vi "GUNSC_LibGetMaxAmps.vi"(8 "error in (no error)":errorcluster) -> (0 "error out":errorcluster, 2 "max amps":i32)   [LabVIEW 2014]
uses:
  public/c/lib/libunsc.so
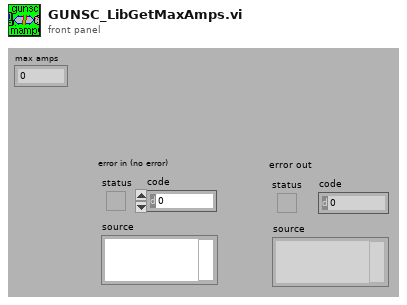
[diagram p1: front panel]
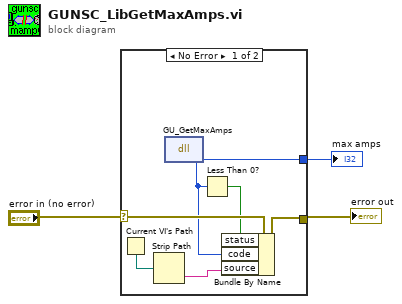
[diagram p0: block diagram]
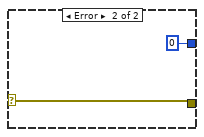
[diagram p2: hidden frame]
diagram:
  n1 = case shown="No Error" "error in (no error)" {
    selector: "error in (no error)" -> [w9 w11]
    tunnel: [w7 0] -> w3
    tunnel: [w4 w11] -> w1
    frame No Error {
      n2 = Current VI's Path() -> (path=w6:path)
      n3 = Strip Path(path=w6) -> (name=w5:string)  [unwired: 1 out]
      n4 = dll-call lib="home/sispi/Panview-1.13.0-64b/PAN/Modules/GUNSC/public/c/lib/libunsc.so" fn="GU_GetMaxAmps"() -> ("return type"=w7:i32)  [unwired: 3 in, 2 out]
      n5 = Less Than 0?(x=w7) -> (x < 0?=w8:bool)
      n6 = Bundle By Name(cluster=w9, "status"=w8, "code"=w7, "source"=w5) -> (w4:errorcluster)
    }
    frame Error {
    }
  }
  "max amps" <- w3
  "error out" <- w1
